vi "Write Destinations.vi"(8 "error in (no error)":errorcluster, 10 "Destinations":string[](array[string]), 11 "SignalManager in":refnum<class "SignalManager.lvclass">) -> (0 "error out":errorcluster, 3 "SignalManager out":refnum<class "SignalManager.lvclass">)   [LabVIEW 2020, in "SignalManager.lvclass"]
uses:
  SignalManager.lvclass
  SignalManager.lvclass/SignalManager.ctl
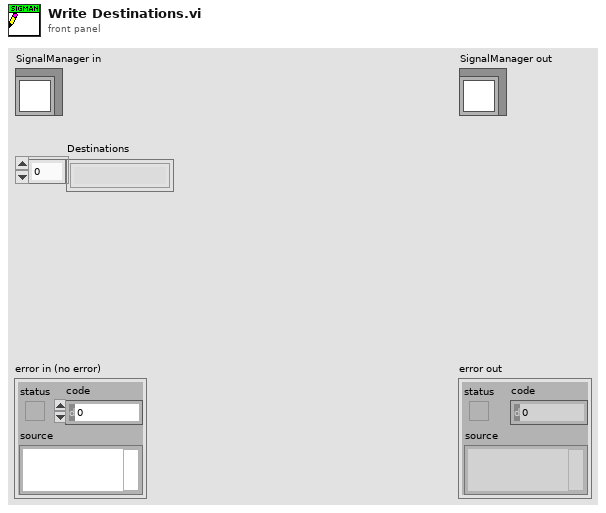
[diagram p1: front panel]
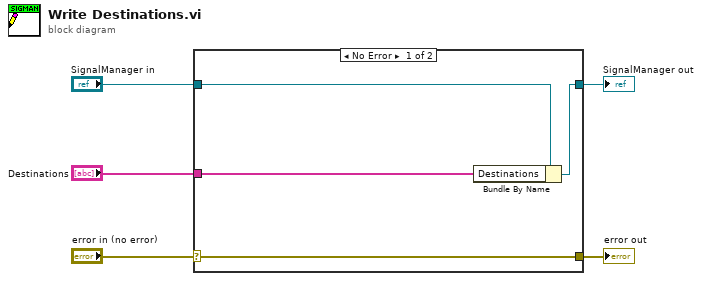
[diagram p0: block diagram]
diagram:
  n1 = case shown="No Error" "error in (no error)" {
    selector: "error in (no error)" -> [w9 w10]
    tunnel: [w9 w10] -> w4
    tunnel: [w7 w11] -> w2
    tunnel: "SignalManager in" -> [w8 w11]
    tunnel: "Destinations" -> [w6 _]
    frame No Error {
      n2 = Bundle By Name(cluster=w8, "Destinations"=w6) -> (w7:refnum<class "SignalManager.lvclass">)
    }
    frame Error {
    }
  }
  "error out" <- w4
  "SignalManager out" <- w2
